vi "Set Name.vi"(7 "Set IP Packet":string, 10 "Input parameter 1":string, 11 "MAC Address HEX":string) -> (3 "Output frame":string)   [LabVIEW 2017]
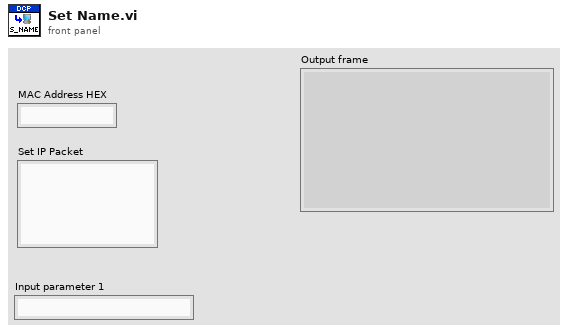
[diagram p1: front panel]
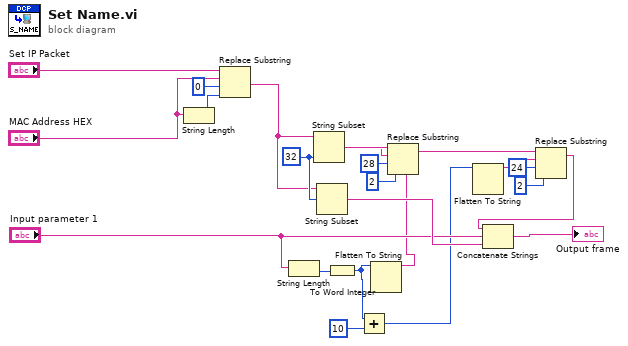
[diagram p0: block diagram]
diagram:
  w18 = 32 ("offset (0)")
  n1 = String Length(string="MAC Address HEX") -> (length=w21:i32)
  n2 = Replace Substring(2:w21, 3:0 ("offset (0)"), 4:"MAC Address HEX", 5:"Set IP Packet") -> (1:w12:string)  [unwired: 1 out]
  n3 = String Length(string="Input parameter 1") -> (length=w9:i32)
  n4 = String Subset(string=w12, length (rest)=w18) -> (substring=w14:string)  [unwired: 1 in]
  n5 = String Subset(string=w12, offset (0)=w18) -> (substring=w17:string)  [unwired: 1 in]
  n6 = To Word Integer(number=w9) -> (16bit integer=w4:i16)
  n7 = Add(x=w4, y=i16 10) -> (x+y=w2:i16)
  n8 = Flatten To String(anything=w4) -> (data string=w10:string)  [unwired: 3 in, 2 out]
  n9 = Replace Substring(2:2 ("length (len. of substring)"), 3:28 ("offset (0)"), 4:w10, 5:w14) -> (1:w8:string)  [unwired: 1 out]
  n10 = Flatten To String(anything=w2) -> (data string=w7:string)  [unwired: 3 in, 2 out]
  n11 = Replace Substring(2:2 ("length (len. of substring)"), 3:24 ("offset (0)"), 4:w7, 5:w8) -> (1:w1:string)  [unwired: 1 out]
  n12 = Concatenate Strings(w1, "Input parameter 1", w17) -> (→"Output frame":string)
